vi "AddControl(s)ToControlStateArray.vi"   [LabVIEW 2019]
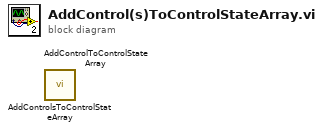
[diagram p0: block diagram]
diagram:
  n1 = call <userlib>:"AddControlsToControlStateArray.vi"() -> ()  [unwired: 10 in, 2 out]
  n2 = call <userlib>:"AddControlToControlStateArray.vi"() -> ()  [unwired: 10 in, 2 out]
